vi "Main ActionVIOnLoad.vi"(8 "error in (no error)":errorcluster, 11 "Device Item Ref in":T1 format="%.0x") -> (0 "error out":errorcluster, 3 "Device Item Ref out":T1 format="%.0x")   [LabVIEW 2014, in "SLSC configuration System Explorer.lvlib"]
uses:
  SLSC configuration System Explorer.lvlib
  <vilib>/NI Veristand/Custom Device API/Custom Device Item Ref.ctl
  <vilib>/NI Veristand/Custom Device API/Custom Device Channel.ctl
  <vilib>/NI Veristand/Custom Device API/Custom Device Channel Type.ctl
  NationalInstruments.VeriStand.SystemDefinitionAPI
  Shared/Constants.vi
  <vilib>/NI Veristand/Custom Device Tools/Custom Device Utility Library/NI VeriStand - Search for All Items by GUID.vi
  <vilib>/NI Veristand/Custom Device API/Set Item Property (U16).vi
  <vilib>/NI Veristand/Custom Device API/Custom Device API.lvlib
  Shared/SLSC configuration Shared.lvlib
  <vilib>/NI Veristand/Custom Device Tools/Custom Device Utility Library/Custom Device Utility Library.lvlib
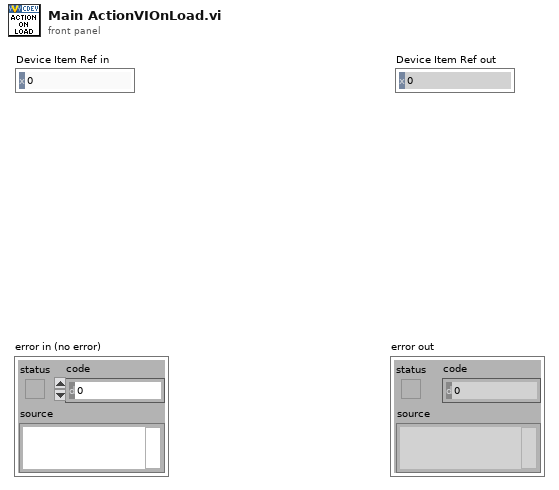
[diagram p1: front panel]
types:
  T1 = typedef "Custom Device API.lvlib/Custom Device Item Ref.ctl" = u64
  T2 = typedef "Custom Device API.lvlib/Custom Device Channel Type.ctl" = enum16{"Input", "Output"}
  T3 = typedef "Custom Device API.lvlib/Custom Device Channel.ctl" = cluster{"Type":T2, "Units":string, "Default Value":dbl, "Faultable":bool, "Scalable":bool}
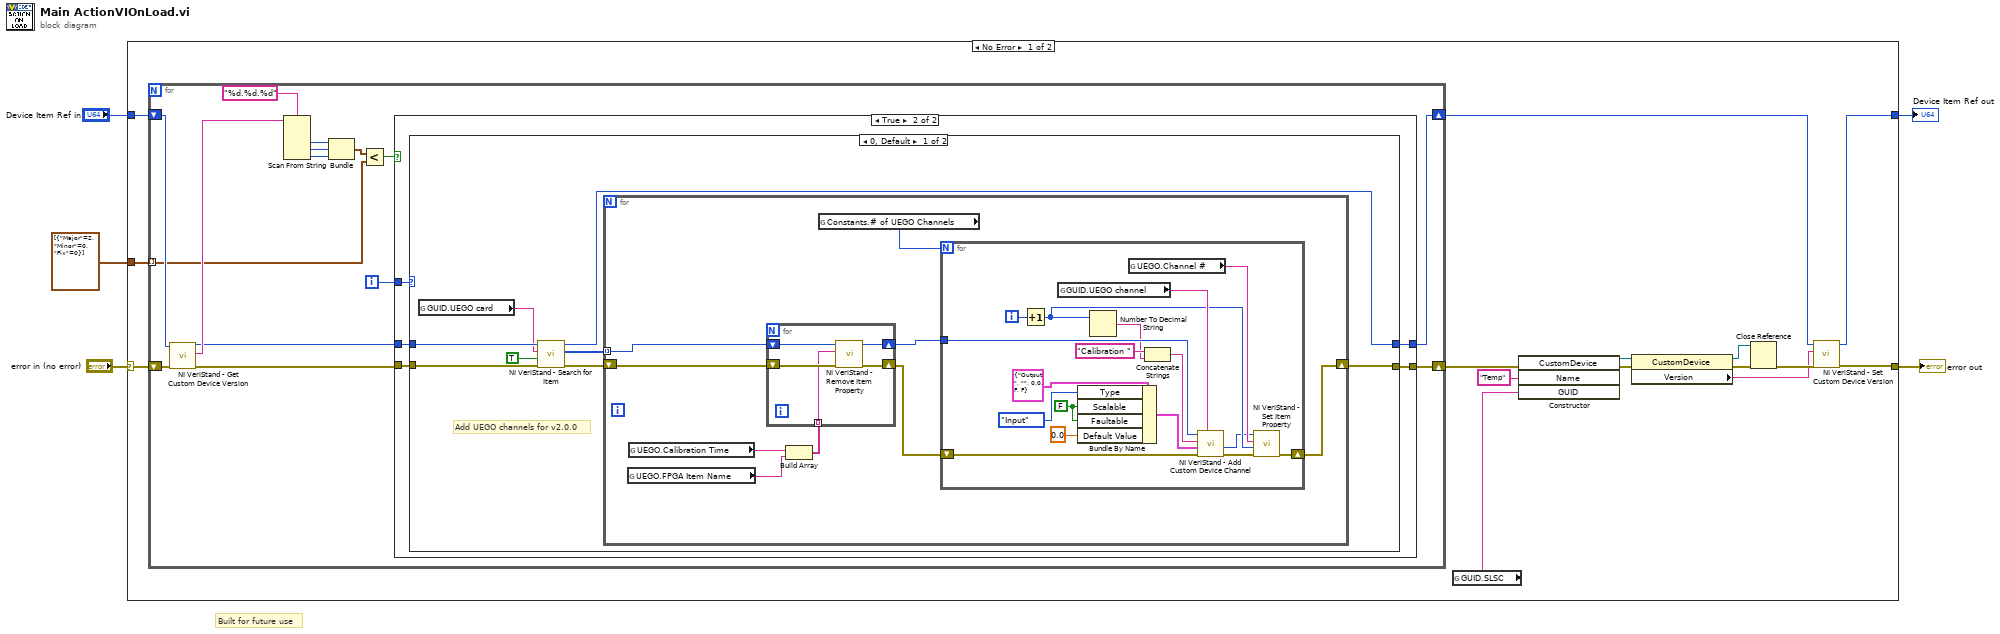
[diagram p0: block diagram]
diagram:
  # "Built for future use"
  n1 = case shown="No Error" "error in (no error)" {
    selector: "error in (no error)" -> [w18 w85]
    tunnel: [w7 w85] -> w2
    tunnel: "Device Item Ref in" -> [w19 w84]
    tunnel: cluster{"Major":i32, "Minor":i32, "Fix":i32}[] [{"Major"=2, "Minor"=0, "Fix"=0}] -> [w20 _]
    tunnel: [w6 w84] -> w1
    frame No Error {
      n2 = for {
        tunnel: w20 -> [w27] mode=indexing
        shift-right: [w21] -> w9
        shift-left: w19 -> [w34]
        shift-right: [w23] -> w17
        shift-left: w18 -> [w35]
        i -> [w25]
        n3 = call <vilib>:"NI VeriStand - Get Custom Device Version.vi"("error in (no error)"=w35, "Device Ref in"=w34) -> ("error out"=w24:errorcluster, "Value"=w32:string, "Device Ref out"=w22:T1)  [unwired: 7 in]
        n4 = Scan From String(format string="%d.%d.%d", input string=w32) -> (output 1=w31:i32, output 2=w30:i32, output 3=w29:i32)  [unwired: 5 in, 3 out]
        n5 = Bundle(w31, w30, w29) -> (w28:cluster{i32, i32, i32})  [unwired: 1 in]
        n6 = Less?(x=w28, y=w27) -> (x < y?=w26:bool)
        n7 = case shown="True" w26 {
          tunnel: w25 -> [_ w42]
          tunnel: w24 -> [w37 w41]
          tunnel: [w37 w40] -> w23
          tunnel: w22 -> [w36 w39]
          tunnel: [w36 w38] -> w21
          frame False {
          }
          frame True {
            n8 = case shown="0, Default" w42 {
              tunnel: w41 -> [w50 w83]
              tunnel: [w44 w83] -> w40
              tunnel: w39 -> [w49 w82]
              tunnel: [w48 w82] -> w38
              frame 0, Default {
                # "Add UEGO channels for v2.0.0"
                n9 = global read "Constants.vi" "GUID.UEGO card"() -> (w46:string)
                n10 = call-poly <vilib>:"NI VeriStand - Search for Item.vi"("error in"=w50, "Find All? (T)"=TRUE, "Item GUID"=w46, "Section Ref in"=w49) -> ("error out"=w45:errorcluster, "Item Refs"=w43:T1[], "Section Ref out"=w48:T1)  [unwired: 4 in, 1 out]
                n11 = for {
                  shift-right: [w58] -> w44
                  shift-left: w45 -> [w57]
                  tunnel: w43 -> [w56] mode=indexing
                  n12 = global read "Constants.vi" "UEGO.FPGA Item Name"() -> (w54:string)
                  n13 = global read "Constants.vi" "UEGO.Calibration Time"() -> (w53:string)
                  n14 = Build Array(w53, w54) -> (w51:string[])
                  n15 = for {
                    shift-right: [w62] -> w55
                    shift-left: w56 -> [w63]
                    shift-right: [w61] -> w52
                    shift-left: w57 -> [w64]
                    tunnel: w51 -> [w60] mode=indexing
                    n16 = call <vilib>:"NI VeriStand - Remove Item Property.vi"("error in (no error)"=w64, "Property Name"=w60, "Item Ref in"=w63) -> ("error out"=w61:errorcluster, "Item Ref out"=w62:T1)  [unwired: 6 in, 1 out]
                  }
                  n17 = global read "Constants.vi" "Constants.# of UEGO Channels"() -> (w59:u8)
                  n18 = for {
                    N: w59 -> [_]
                    shift-right: [w67] -> w58
                    shift-left: w52 -> [w79]
                    tunnel: w55 -> [w78]
                    i -> [w80]
                    w71 = FALSE ("Scalable")
                    n19 = Increment(x=w80) -> (x+1=w66:i32)
                    n20 = global read "Constants.vi" "GUID.UEGO channel"() -> (w68:string)
                    n21 = Bundle By Name(cluster=T3 {"Type"=enum."Output", "Units"="", "Default Value"=0.0, "Faultable"=FALSE, "Scalable"=FALSE} ("Channel"), "Type"=Custom_Device_Channel_Type."Input", "Scalable"=w71, "Faultable"=w71, "Default Value"=0.0) -> (w69:T3)
                    n22 = Number To Decimal String(number=w66) -> (decimal integer string=w75:string)  [unwired: 1 in]
                    n23 = global read "Constants.vi" "UEGO.Channel #"() -> (w81:string)
                    n24 = Concatenate Strings("Calibration " ("Channel Name"), w75) -> (w74:string)
                    n25 = call <vilib>:"NI VeriStand - Add Custom Device Channel.vi"("GUID (Default Channel)"=w68, "error in (no error)"=w79, "Channel"=w69, "Channel Name"=w74, "Parent Ref in"=w78) -> ("error out"=w77:errorcluster, "Channel Ref"=w65:T1)  [unwired: 3 in, 2 out]
                    n26 = call-poly <vilib>:"NI VeriStand - Set Item Property.vi"("error in (no error)"=w77, "Value"=w66, "Property Name"=w81, "Item Ref in"=w65) -> ("error out"=w67:errorcluster)  [unwired: 5 in, 2 out]
                  }
                }
              }
              frame 1 {
              }
            }
          }
        }
      }
      n27 = global read "Constants.vi" "GUID.SLSC"() -> (w15:string)
      n28 = constructor class="CustomDevice"(error in=w17, "Name"="Temp", "GUID"=w15) -> (reference out=w13:refnum<k24>, error out=w14:errorcluster)  [unwired: 2 in, 3 out]
      n29 = property class="CustomDevice"(reference=w13, error in=w14) -> (reference out=w11:refnum<k24>, error out=w12:errorcluster, "Version"=w8:string)
      n30 = Close Reference(reference=w11, error in (no error)=w12) -> (error out=w10:errorcluster)
      n31 = call <vilib>:"NI VeriStand - Set Custom Device Version.vi"("error in (no error)"=w10, "Value"=w8, "Device Ref in"=w9) -> ("error out"=w7:errorcluster, "Device Ref out"=w6:T1)  [unwired: 7 in]
    }
    frame Error {
    }
  }
  "error out" <- w2
  "Device Item Ref out" <- w1
